vi "xDaqinfo Cluster to XML.vi"(1 "DAQ Info Cluster":T1={"Data Chunks per File"=1000, "Samples per Waveform"=95, "Pretrigger Samples"=15, "circular buffer length (samples)"=1000, "Waveforms per Data Chunk"=5000} {"Waveforms per Data Chunk" format="%.2p"}, 2 "Input String":string) -> (0 "Output String":string)   [LabVIEW 2014]
panel:
  # "Waveform/Data Chunk information"
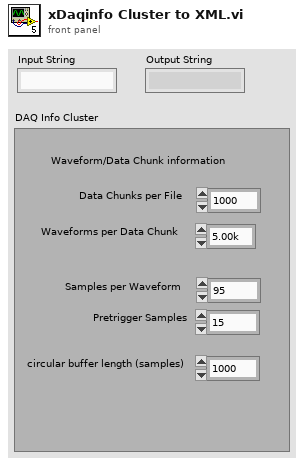
[diagram p1: front panel]
types:
  T1 = cluster{"Data Chunks per File":u32, "Samples per Waveform":u32, "Pretrigger Samples":u32, "circular buffer length (samples)":u32, "Waveforms per Data Chunk":u32}
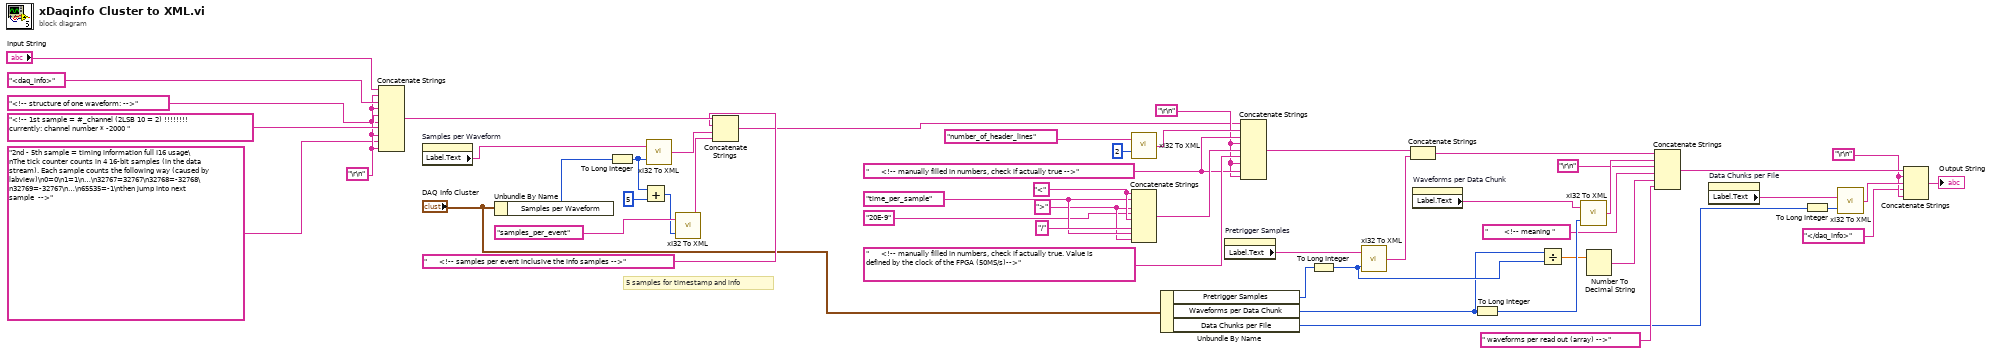
[diagram p0: block diagram]
diagram:
  w11 = "\r\n"
  w33 = ">" ("string")
  w36 = "<" ("string")
  w34 = "time_per_sample" ("variable name")
  w29 = "      <!-- manually filled in numbers, check if actually true -->" ("string")
  w28 = "\r\n"
  w46 = "\r\n"
  # "5 samples for timestamp and info"
  n1 = Concatenate Strings("Input String", w46, "<daq_info>" ("string"), w46, "<!-- structure of one waveform: -->", w46, "<!-- 1st sample = #_channel (2LSB 10 = 2) !!!!!!!! currently: channel number * -2000 " ("string"), w46, "2nd - 5th sample = timing information full I16 usage\nThe tick counter counts in 4 16-bit samples (in the data stream). Each sample counts the following way (caused by labview)\n0=0\n1=1\n…\n32767=32767\n32768=-32768\n32769=-32767\n…\n65535=-1\nthen jump into next sample  -->" ("string"), w46) -> (w43:string)
  n2 = property on="Samples per Waveform" class="DigNum (strict)"() -> ("Label.Text"=w4:string)  [unwired: 2 in, 2 out]
  n3 = Unbundle By Name("DAQ Info Cluster") -> ("Samples per Waveform"=w9:u32)
  n4 = To Long Integer(number=w9) -> (32bit integer=w49:i32)
  n5 = Add(x=w49, y=5) -> (x+y=w47:i32)
  n6 = call "xI32 To XML.vi"("variable"=w49, "variable name"=w4) -> ("xml string"=w45:string)
  n7 = call "xI32 To XML.vi"("variable"=w47, "variable name"="samples_per_event") -> ("xml string"=w44:string)
  n8 = Concatenate Strings(w43, "      <!-- samples per event inclusive the info samples -->" ("string"), w45, w44) -> (w14:string)
  n9 = call "xI32 To XML.vi"("variable"=2, "variable name"="number_of_header_lines") -> ("xml string"=w39:string)
  n10 = Concatenate Strings(w36, w34, w33, "20E-9" ("string"), w36, "/" ("string"), w34, w33) -> (w31:string)
  n11 = Unbundle By Name("DAQ Info Cluster") -> ("Pretrigger Samples"=w8:u32, "Waveforms per Data Chunk"=w7:u32, "Data Chunks per File"=w6:u32)
  n12 = property on="Pretrigger Samples" class="DigNum (strict)"() -> ("Label.Text"=w2:string)  [unwired: 2 in, 2 out]
  n13 = Concatenate Strings(w14, w39, w29, w28, w31, "      <!-- manually filled in numbers, check if actually true. Value is defined by the clock of the FPGA (50MS/s)-->" ("string"), w28, w29, w28) -> (w19:string)
  n14 = To Long Integer(number=w8) -> (32bit integer=w24:i32)
  n15 = call "xI32 To XML.vi"("variable"=w24, "variable name"=w2) -> ("xml string"=w20:string)
  n16 = Concatenate Strings(w19, w20) -> (w13:string)
  n17 = property on="Waveforms per Data Chunk" class="DigNum (strict)"() -> ("Label.Text"=w3:string)  [unwired: 2 in, 2 out]
  n18 = To Long Integer(number=w7) -> (32bit integer=w22:i32)
  n19 = Divide(x=w7, y=w24) -> (x/y=w21:dbl)
  n20 = call "xI32 To XML.vi"("variable"=w22, "variable name"=w3) -> ("xml string"=w23:string)
  n21 = Number To Decimal String(number=w21) -> (decimal integer string=w16:string)  [unwired: 1 in]
  n22 = Concatenate Strings(w13, w23, "\r\n", "        <!-- meaning " ("string"), w16, " waveforms per read out (array) -->" ("string")) -> (w27:string)
  n23 = property on="Data Chunks per File" class="DigNum (strict)"() -> ("Label.Text"=w1:string)  [unwired: 2 in, 2 out]
  n24 = To Long Integer(number=w6) -> (32bit integer=w25:i32)
  n25 = call "xI32 To XML.vi"("variable"=w25, "variable name"=w1) -> ("xml string"=w26:string)
  n26 = Concatenate Strings(w27, w11, w26, "</daq_info>" ("string"), w11) -> (→"Output String":string)
